vi "Finish.vi"   [LabVIEW 2016]
doc: "This VI is called just before exiting. It is expected to close I/O refnum, save collected data, etc."
uses:
  <vilib>/Rock Robotics/WPI/Utilities/WPI_GetSetVariantRefNum.vi
types:
  T1 = typedef "WPI_MotorControlDeviceRef.ctl" = cluster{"DeviceStatus":errorcluster, "Type":T2, "PWM":cluster{"PWM Channel":T3, "DeadBand":T4}, "CAN":cluster{"Device Number":u8, "SetOutput VI Ref":variant, "GetOutput VI Ref":variant, "Enable VI Ref":variant, "Disable VI Ref":variant, "Data":variant}, "Invert":bool}
  T2 = typedef "WPI_MotorControlType.ctl" = enum16{"PWM", "CAN"}
  T3 = typedef "FPGA_DIOPWMChannel.ctl" = enum8{"PWM 0", "PWM 1", "PWM 2", "PWM 3", "PWM 4", "PWM 5", "PWM 6", "PWM 7", "PWM 8", "PWM 9", "PWM MXP 0", "PWM MXP 1", "PWM MXP 2", "PWM MXP 3", "PWM MXP 4", "PWM MXP 5", "PWM MXP 6", "PWM MXP 7", "PWM MXP 8", "PWM MXP 9", "Invalid"}
  T4 = typedef "WPI_PWMDeadband.ctl" = cluster{"Name":string, "maxPositivePwm":i32, "minPositivePwm":i32, "centerPwm":i32, "maxNegativePwm":i32, "minNegativePwm":i32, "angularRange":u16}
  T5 = typedef "WPI_DigitalInputDevRef.ctl" = cluster{"DevStatus":errorcluster, "DIO Channel":T6}
  T6 = typedef "FPGA_DIOChannel.ctl" = enum8{"DIO 0", "DIO 1", "DIO 2", "DIO 3", "DIO 4", "DIO 5", "DIO 6", "DIO 7", "DIO 8", "DIO 9", "DIO MXP 0", "DIO MXP 1", "DIO MXP 2", "DIO MXP 3", "DIO MXP 4", "DIO MXP 5", "DIO MXP 6", "DIO MXP 7", "DIO MXP 8", "DIO MXP 9", "DIO MXP 10", "DIO MXP 11", "DIO MXP 12", "DIO MXP 13", "DIO MXP 14", "DIO MXP 15", "SPI Port CS1", "SPI Port CS2", "SPI Port CS3", "SPI Port MISO", "SPI Port MOSI", "Invalid"}
  T7 = typedef "WPI_JoystickDevRef.ctl" = cluster{"Device":T8}
  T8 = typedef "WPI_JoystickDeviceEnum.ctl" = enum16{"USB 0", "USB 1", "USB 2", "USB 3", "USB 4", "USB 5"}
  T9 = typedef "WPI_RobotDriveDevRef.ctl" = cluster{"DevStatus":errorcluster, "Motors[]":T1[], "Square Inputs":bool, "Max Output":dbl}
  T10 = typedef "WPI_ServoDeviceRef.ctl" = cluster{"DeviceStatus":errorcluster, "PWM Channel":T3, "DeadBand":T4}
  T11 = typedef "WPI_GyroDevRef.ctl" = cluster{"DevStatus":errorcluster, "Analog Channel":T12, "Offset":dbl, "Gain (VoltsPerDegree/Second)":dbl, "Gyro Type":enum16{"Analog", "XRS450"}, "Handle":i32, "SPI Bus":T13, "Device Found":bool, "Sample Rate":dbl, "Calibrate On Open":bool}
  T12 = typedef "FPGA_AIChannel.ctl" = enum8{"AI 0", "AI 1", "AI 2", "AI 3", "AI MXP 0", "AI MXP 1", "AI MXP 2", "AI MXP 3", "Invalid"}
  T13 = typedef "spi_bus.ctl" = enum16{"SPI On-Board, CS0", "SPI On-Board, CS1", "SPI On-Board, CS2", "SPI On-Board, CS3", "SPI MXP", "Invalid"}
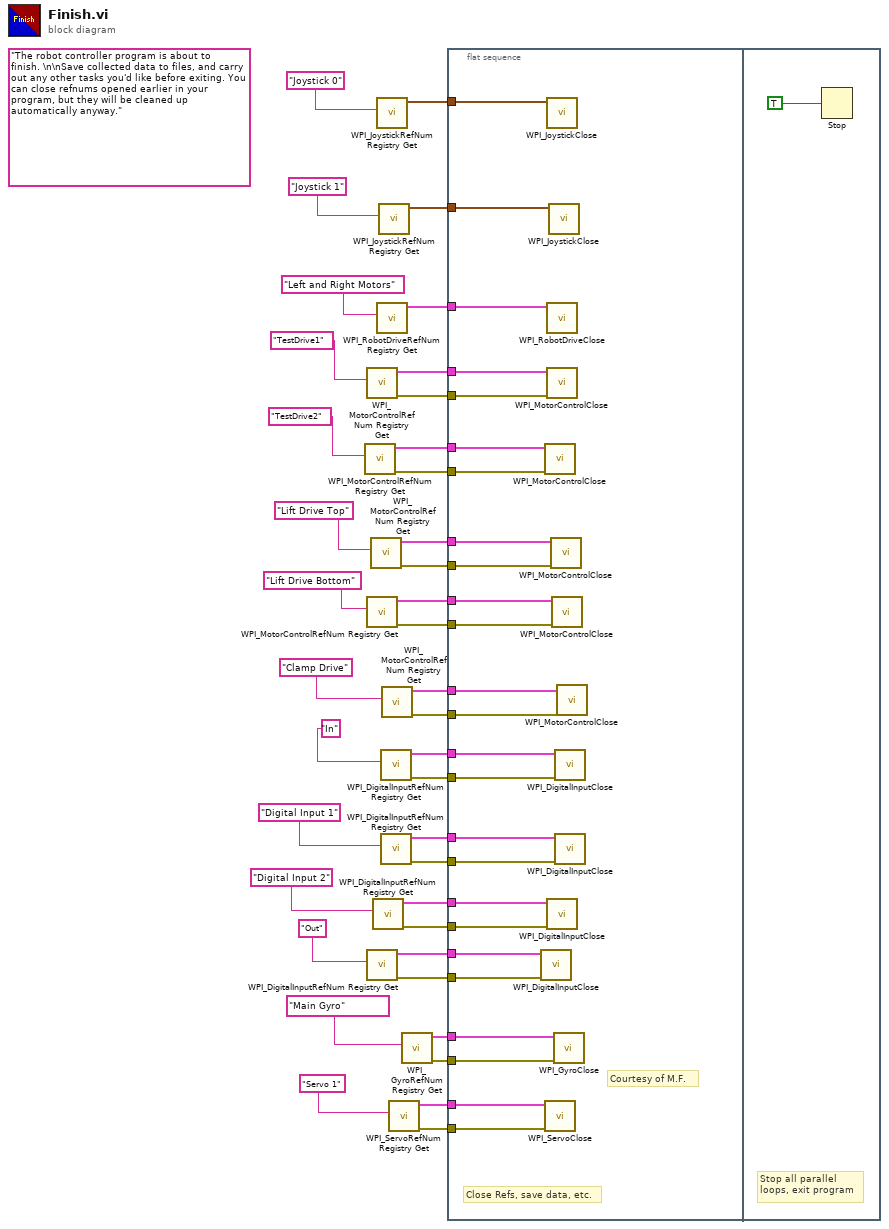
[diagram p0: block diagram]
diagram:
  (unwired) "The robot controller program is about to finish. \n\nSave collected data to files, and carry out any other tasks you'd like before exiting. You can close refnums opened earlier in your program, but they will be cleaned up automatically anyway."
  n1 = call <vilib>:"WPI_MotorControlRefNum Registry Get.vi"("refnum name"="TestDrive2") -> ("error out"=w1:errorcluster, "MotorControlDevRef"=w2:T1)  [unwired: 9 in]
  n2 = call <vilib>:"WPI_MotorControlRefNum Registry Get.vi"("refnum name"="TestDrive1") -> ("error out"=w6:errorcluster, "MotorControlDevRef"=w5:T1)  [unwired: 9 in]
  n3 = call <vilib>:"WPI_MotorControlRefNum Registry Get.vi"("refnum name"="Lift Drive Bottom") -> ("error out"=w23:errorcluster, "MotorControlDevRef"=w24:T1)  [unwired: 9 in]
  n4 = call <vilib>:"WPI_DigitalInputRefNum Registry Get.vi"("refnum name"="Out") -> ("error out"=w13:errorcluster, "DigitalInputDevRef"=w14:T5)  [unwired: 9 in]
  n5 = call <vilib>:"WPI_MotorControlRefNum Registry Get.vi"("refnum name"="Lift Drive Top") -> ("error out"=w25:errorcluster, "MotorControlDevRef"=w26:T1)  [unwired: 9 in]
  n6 = call <vilib>:"WPI_DigitalInputRefNum Registry Get.vi"("refnum name"="Digital Input 2") -> ("error out"=w15:errorcluster, "DigitalInputDevRef"=w16:T5)  [unwired: 9 in]
  n7 = call <vilib>:"WPI_JoystickRefNum Registry Get.vi"("refnum name"="Joystick 0") -> ("JoystickDevRef"=w36:T7)  [unwired: 1 in, 9 out]
  n8 = call <vilib>:"WPI_RobotDriveRefNum Registry Get.vi"("refnum name"="Left and Right Motors") -> ("RobotDriveDevRef"=w37:T9)  [unwired: 1 in, 9 out]
  n9 = call <vilib>:"WPI_JoystickRefNum Registry Get.vi"("refnum name"="Joystick 1") -> ("JoystickDevRef"=w8:T7)  [unwired: 1 in, 9 out]
  n10 = call <vilib>:"WPI_DigitalInputRefNum Registry Get.vi"("refnum name"="In") -> ("error out"=w19:errorcluster, "DigitalInputDevRef"=w20:T5)  [unwired: 9 in]
  n11 = call <vilib>:"WPI_DigitalInputRefNum Registry Get.vi"("refnum name"="Digital Input 1") -> ("error out"=w17:errorcluster, "DigitalInputDevRef"=w18:T5)  [unwired: 9 in]
  n12 = call <vilib>:"WPI_MotorControlRefNum Registry Get.vi"("refnum name"="Clamp Drive") -> ("error out"=w21:errorcluster, "MotorControlDevRef"=w22:T1)  [unwired: 9 in]
  n13 = call <vilib>:"WPI_ServoRefNum Registry Get.vi"("refnum name"="Servo 1") -> ("error out"=w9:errorcluster, "ServoDeviceRef"=w10:T10)  [unwired: 9 in]
  n14 = call <vilib>:"WPI_GyroRefNum Registry Get.vi"("refnum name"="Main Gyro") -> ("error out"=w11:errorcluster, "GyroDevRef"=w12:T11)  [unwired: 9 in]
  n15 = flat-sequence {
    tunnel: w37 -> [w64]
    tunnel: w36 -> [w63]
    tunnel: w26 -> [w62]
    tunnel: w25 -> [w61]
    tunnel: w24 -> [w60]
    tunnel: w23 -> [w59]
    tunnel: w22 -> [w58]
    tunnel: w21 -> [w57]
    tunnel: w20 -> [w56]
    tunnel: w19 -> [w55]
    tunnel: w18 -> [w54]
    tunnel: w17 -> [w53]
    tunnel: w16 -> [w52]
    tunnel: w15 -> [w51]
    tunnel: w14 -> [w50]
    tunnel: w13 -> [w49]
    tunnel: w12 -> [w48]
    tunnel: w11 -> [w47]
    tunnel: w10 -> [w46]
    tunnel: w9 -> [w45]
    tunnel: w8 -> [w44]
    tunnel: w5 -> [w42]
    tunnel: w6 -> [w43]
    tunnel: w2 -> [w41]
    tunnel: w1 -> [w40]
    frame #0 {
      # "Courtesy of M.F."
      # "Close Refs, save data, etc."
      n16 = call <vilib>:"WPI_DigitalInputClose.vi"("error in (no error)"=w49, "DigitalInputDevRef"=w50) -> ()  [unwired: 9 in, 1 out]
      n17 = call <vilib>:"WPI_MotorControlClose.vi"("error in"=w40, "MotorControlDevRef"=w41) -> ()  [unwired: 9 in, 1 out]
      n18 = call <vilib>:"WPI_ServoClose.vi"("error in (no error)"=w45, "ServoDeviceRef"=w46) -> ()  [unwired: 9 in, 1 out]
      n19 = call <vilib>:"WPI_JoystickClose.vi"("JoystickDevRef"=w63) -> ()  [unwired: 11 out]
      n20 = call <vilib>:"WPI_RobotDriveClose.vi"("RobotDriveDevRef"=w64) -> ()  [unwired: 1 in, 10 out]
      n21 = call <vilib>:"WPI_MotorControlClose.vi"("error in"=w43, "MotorControlDevRef"=w42) -> ()  [unwired: 9 in, 1 out]
      n22 = call <vilib>:"WPI_DigitalInputClose.vi"("error in (no error)"=w51, "DigitalInputDevRef"=w52) -> ()  [unwired: 9 in, 1 out]
      n23 = call <vilib>:"WPI_JoystickClose.vi"("JoystickDevRef"=w44) -> ()  [unwired: 11 out]
      n24 = call <vilib>:"WPI_MotorControlClose.vi"("error in"=w61, "MotorControlDevRef"=w62) -> ()  [unwired: 9 in, 1 out]
      n25 = call <vilib>:"WPI_MotorControlClose.vi"("error in"=w59, "MotorControlDevRef"=w60) -> ()  [unwired: 9 in, 1 out]
      n26 = call <vilib>:"WPI_GyroClose.vi"("error in"=w47, "GyroDevRef"=w48) -> ()  [unwired: 9 in, 1 out]
      n27 = call <vilib>:"WPI_DigitalInputClose.vi"("error in (no error)"=w55, "DigitalInputDevRef"=w56) -> ()  [unwired: 9 in, 1 out]
      n28 = call <vilib>:"WPI_DigitalInputClose.vi"("error in (no error)"=w53, "DigitalInputDevRef"=w54) -> ()  [unwired: 9 in, 1 out]
      n29 = call <vilib>:"WPI_MotorControlClose.vi"("error in"=w57, "MotorControlDevRef"=w58) -> ()  [unwired: 9 in, 1 out]
    }
    frame #1 {
      # "Stop all parallel\nloops, exit program"
      n30 = Stop(stop? (T)=TRUE ("Quit")) -> ()
    }
  }
